vi "Set Enum String Value_csm.vi"(8 "error in (no error)":errorcluster, 9 "String Value":string, 10 "Default Enum Value":variant) -> (0 "error out":errorcluster, 2 "Enum":variant)   [LabVIEW 2017, in "Communicable State Machine.lvlib"]
doc: "Sets an enum's integer value to the position within the enum's strings matching the <B>String Value</B> input. Returns<B> Default Enum Value</B> if an error occurs."
uses:
  Communicable State Machine.lvlib
panel:
  # "[OpenG VI Tags] ***Do Not Remove***"
  # "Set Enum String Value.vi\n\nSets an enum's integer value to the position within the enum's strings matching \n\nPlease visit http://www.OpenG.org to learn about the\nOpen Source LabVIEW software movement.\n\nNOTICE -- YOU MUST LEAVE THIS NOTICE IN PLACE.  PER THE TERMS OF THE LICENSE BELOW, YOU MAY SUBLICENSE THIS SOFTWARE \nIN ANY WAY THAT DOES NOT CONFLICT WITH THIS LICENSE.\n\n### BSD License (http://www.opensource.org/licenses/bsd-license.php) Begin ###\n \nCopyright (c) 2002, Jean-Pierre Drolet <drolet_jp@hotmail.com>\nCopyright (c) 2002-2006, Jim Kring <jim@jimkring.com>\n\nAll rights reserved.\n\nRedistribution and use in source and binary forms, with or without modification, are permitted provided that the following conditions are met:\n\n    * Redistributions of source code must retain the above copyright notice, this list of conditions and the following disclaimer.\n    * Redistributions in binary form must reproduce the above copyright notice, this list of conditions and the following disclaimer in the \n       documentation and/or other materials provided with the distribution.\n    * Neither the name of SciWare, James Kring, Inc., nor the names of its contributors may be used to endorse or promote products derived \n       from this software without specific prior written permission.\n\nTHIS SOFTWARE IS PROVIDED BY THE COPYRIGHT HOLDERS AND CONTRIBUTORS \"AS IS\" AND ANY EXPRESS OR IMPLIED WARRANTIES, \nINCLUDING, BUT NOT LIMITED TO, THE IMPLIED WARRANTIES OF MERCHANTABILITY AND FITNESS FOR A PARTICULAR PURPOSE ARE \nDISCLAIMED. IN NO EVENT SHALL THE COPYRIGHT OWNER OR CONTRIBUTORS BE LIABLE FOR ANY DIRECT, INDIRECT, INCIDENTAL,\n SPECIAL, EXEMPLARY, OR CONSEQUENTIAL DAMAGES (INCLUDING, BUT NOT LIMITED TO, PROCUREMENT OF SUBSTITUTE GOODS OR \nSERVICES; LOSS OF USE, DATA, OR PROFITS; OR BUSINESS INTERRUPTION) HOWEVER CAUSED AND ON ANY THEORY OF LIABILITY, \nWHETHER IN CONTRACT, STRICT LIABILITY, OR TORT (INCLUDING NEGLIGENCE OR OTHERWISE) ARISING IN ANY WAY OUT OF THE USE \nOF THIS SOFTWARE, EVEN IF ADVISED OF THE POSSIBILITY OF SUCH DAMAGE.\n\n### BSD License End ###"
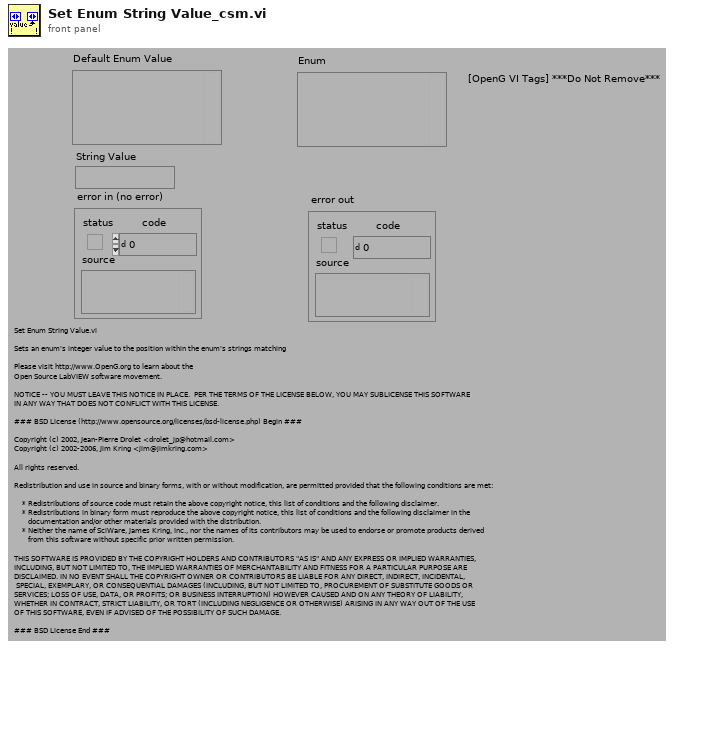
[diagram p1: front panel]
types:
  T1 = cluster{"length":u16, "private":u8, "type":enum8{"<Null>", "I8", "I16", "I32", "I64", "U8", "U16", "U32", "U64", "SGL", "DBL", "EXT", "CSG", "CDB", "CXT", "0x0F", "0x10", "0x11", "0x12", "0x13", "0x14", "Enum U8", "Enum U16", "Enum U32", "Enum U64", "SGL PQ", "DBL PQ", "EXT PQ", "CSG PQ", "CDB PQ", "CXT PQ", "0x1F", "0x20", "Boolean", "0x22", "0x23", "0x24", "0x25", "0x26", "0x27", "0x28", "0x29", "0x2A", "0x2B", "0x2C", "0x2D", "0x2E", "0x2F", "String", "0x31", "Path", "Pict", "0x34", "0x35", "0x36", "DAQ", "0x38", "0x39", "0x3A", "0x3B", "0x3C", "0x3D", "0x3E", "0x3F", "Array", "0x41", "0x42", "0x43", "0x44", "0x45", "0x46", "0x47", "0x48", "0x49", "0x4A", "0x4B", "0x4C", "0x4D", "0x4E", "0x4F", "Cluster", "0x51", "0x52", "Variant", "Waveform", "0x55", "0x56", "0x57", "0x58", "0x59", "0x5A", "0x5B", "0x5C", "0x5D", "0x5E", "Fixed Point", "0x60", "0x61", "0x62", "0x63", "0x64", "0x65", "0x66", "0x67", "0x68", "0x69", "0x6A", "0x6B", "0x6C", "0x6D", "0x6E", "0x6F", "Refnum", "0x71", "0x72", "Set Collection", "Map Collection"}, "# elements":u16}
  T2 = enum8{"<Null>", "I8", "I16", "I32", "I64", "U8", "U16", "U32", "U64", "SGL", "DBL", "EXT", "CSG", "CDB", "CXT", "0x0F", "0x10", "0x11", "0x12", "0x13", "0x14", "Enum U8", "Enum U16", "Enum U32", "Enum U64", "SGL PQ", "DBL PQ", "EXT PQ", "CSG PQ", "CDB PQ", "CXT PQ", "0x1F", "0x20", "Boolean", "0x22", "0x23", "0x24", "0x25", "0x26", "0x27", "0x28", "0x29", "0x2A", "0x2B", "0x2C", "0x2D", "0x2E", "0x2F", "String", "0x31", "Path", "Pict", "0x34", "0x35", "0x36", "DAQ", "0x38", "0x39", "0x3A", "0x3B", "0x3C", "0x3D", "0x3E", "0x3F", "Array", "0x41", "0x42", "0x43", "0x44", "0x45", "0x46", "0x47", "0x48", "0x49", "0x4A", "0x4B", "0x4C", "0x4D", "0x4E", "0x4F", "Cluster", "0x51", "0x52", "Variant", "Waveform", "0x55", "0x56", "0x57", "0x58", "0x59", "0x5A", "0x5B", "0x5C", "0x5D", "0x5E", "Fixed Point", "0x60", "0x61", "0x62", "0x63", "0x64", "0x65", "0x66", "0x67", "0x68", "0x69", "0x6A", "0x6B", "0x6C", "0x6D", "0x6E", "0x6F", "Refnum", "0x71", "0x72", "Set Collection", "Map Collection"}
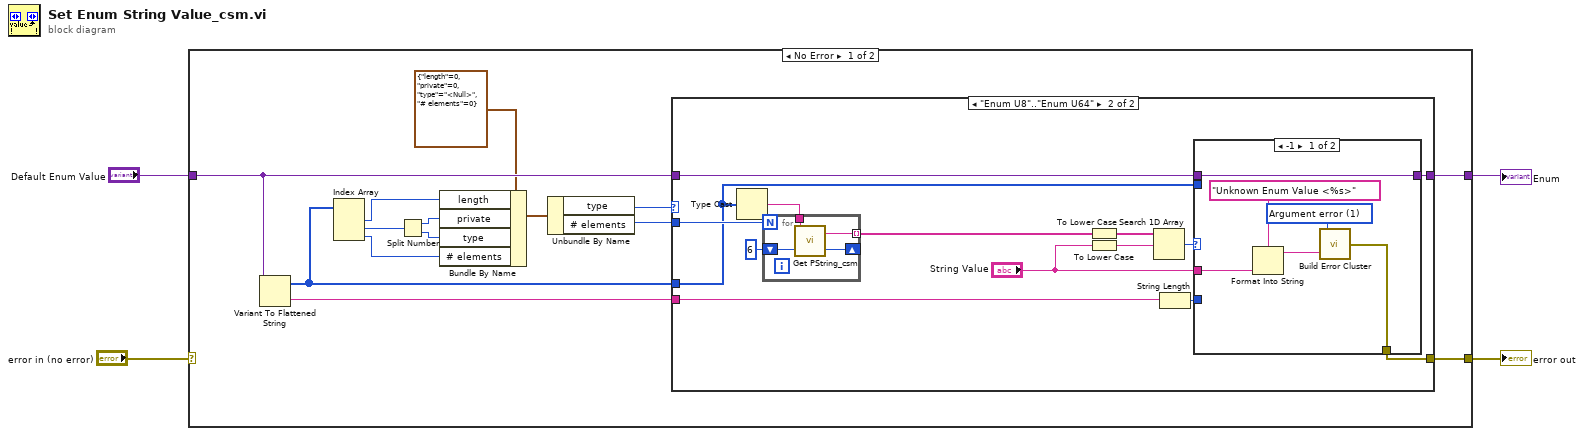
[diagram p0: block diagram]
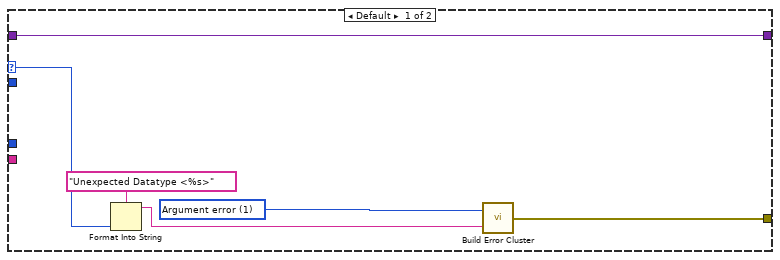
[diagram p2: hidden frame]
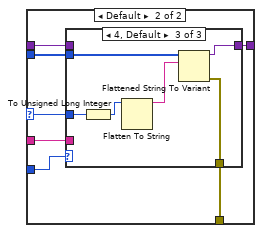
[diagram p3: hidden frame]
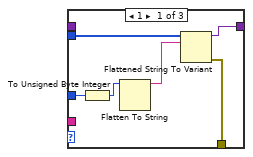
[diagram p4: hidden frame]
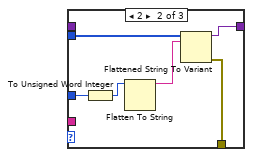
[diagram p5: hidden frame]
diagram:
  n1 = case shown="No Error" "error in (no error)" {
    selector: "error in (no error)" -> [_ w75]
    tunnel: [w18 w75] -> w4
    tunnel: [w12 w74] -> w2
    tunnel: "Default Enum Value" -> [w11 w74]
    frame No Error {
      n2 = Variant To Flattened String(Variant=w11) -> (data string=w14:string, 1:w15:i16[])
      n3 = Index Array(array=w15) -> (element #1=w6:i16, element #2=w9:i16, element #3=w10:i16)  [unwired: 3 in]
      n4 = Split Number(x=w9) -> (hi(x)=w7:u8, lo(x)=w8:u8)
      n5 = Bundle By Name(cluster=T1 {"length"=0, "private"=0, "type"=enum."<Null>", "# elements"=0} ("Type Descriptor Header"), "length"=w6, "private"=w7, "type"=w8, "# elements"=w10) -> (w17:T1)
      n6 = Unbundle By Name(w17) -> ("type"=w16:T2, "# elements"=w13:u16)
      n7 = case shown="\"Enum U8\"..\"Enum U64\"" w16 {
        selector: w16 -> [w21 _]
        tunnel: [w24 w29] -> w18
        tunnel: w15 -> [_ w30]
        tunnel: w14 -> [_ w33]
        tunnel: w13 -> [_ w36]
        tunnel: [w22 w31] -> w12
        tunnel: w11 -> [w22 w32]
        frame Default {
          w23 = 1 items=["No error", "Argument error", "Memory is full", "Out of zone", "End of file", "File already open", "Generic file I/O error", "File not found", "File permission error", "Disk is full", "Duplicate path", "Too many files open", "System feature not enabled", "Resource file not found", "Cannot add resource", "Resource not found", "Image not found", "Image memory error", "Pen does not exist", "Config type invalid", "Config token not found", "Config parse error", "Config memory error", "Bad external code format", "Bad external code offset", "External code not present", "Null window", "Destroy window error", "Null menu", "Print aborted", "Bad print record", "Print driver error", "Windows error during printing", "Memory error during printing", "Print dialog error", "Generic print error", "Invalid device refnum", "Device not found", "Device parameter error", "Device unit error", "Cannot open device", "Device call aborted", "Generic error", "Cancelled by user", "Object ID too low", "Object ID too high", "Object not in heap", "Unknown heap", "Unknown object (invalid DefProc)", "Unknown object (DefProc not in table)", "Message out of range", "Invalid (null) method", "Unknown message", "Manager call not supported", "Bad address", "Network operation in progress", "Network operation timed out", "Connection is busy", "Network attribute not supported", "Network error", "Address in use", "System out of memory", "Connection aborted", "Connection refused", "Not connected", "Already connected", "Connection closed", "Initialization error (interapplication manager)", "Bad occurrence", "Wait on unbound occurrence handler", "Occurrence queue overflow", "Datalog type conflict", "Unused", "Unrecognized type (interapplication manager)", "Memory corrupt", "Failed to make temporary DLL", "Old CIN version", "Drag socket not found", "Failed to load drop-object", "Failed to register OLE object", "Failed to release OLE object", "Format specifier type mismatch", "Unknown format specifier", "Too few format specifiers", "Too many format specifiers", "Scan failed", "Newer CIN version", "Error converting to variant", "Runtime menu error", "Password tampered", "Variant attribute not found", "Incompatible variant data type", "Event data is not available", "Event Store is not present", "Occurrence is not found", "Event Queue is not created", "Event info is not available", "Refnum passed is NULL", "Error retrieving Class GUID", "Error retrieving CoClass GUID", "Error retrieving TypeLib GUID.", "Bad built application magic bytes.", "Specific driver is different from the specific driver associated with the Logical Name.", "There is no session opened to the class driver.", "Max Error", "MAX - Error with config objects", "MAX - Error loading configuration", "MAX - Group not supported"]
          n8 = Format Into String(format string="Unexpected Datatype <%s>" ("Format String"), w21) -> (resulting string=w19:string)  [unwired: 2 in, 1 out]
          n9 = call "Build Error Cluster.vi"("String to Prepend to Source (\"\")"=w19, "Code"=w23) -> ("error out"=w24:errorcluster)
        }
        frame "Enum U8".."Enum U64" {
          n10 = Type Cast(x=w30) -> (*(type *) &x=w35:string)  [unwired: 1 in]
          n11 = for {
            N: w36 -> [_]
            tunnel: w35 -> [w71]
            shift-right: [w72] -> _
            shift-left: 6 -> [w73]
            tunnel: [w70] -> w34 mode=indexing
            n12 = call "Get PString_csm.vi"("Offset (0)"=w73, "String"=w71) -> ("Offset Past PString"=w72:i32, "PString"=w70:string)
          }
          n13 = To Lower Case(string=w34) -> (all lower case string=w25:string[])
          n14 = To Lower Case(string="String Value") -> (all lower case string=w26:string)
          n15 = Search 1D Array(1D array=w25, element=w26) -> (index of element=w27:i32)  [unwired: 1 in]
          n16 = String Length(string=w33) -> (length=w37:i32)
          n17 = case shown="-1" w27 {
            selector: w27 -> [_ w45]
            tunnel: w37 -> [_ w51]
            tunnel: w32 -> [w44 w50]
            tunnel: [w44 w49] -> w31
            tunnel: w30 -> [_ w48]
            tunnel: [w39 w47] -> w29
            tunnel: "String Value" -> [w40 w46]
            frame -1 {
              w43 = 1 items=["No error", "Argument error", "Memory is full", "Out of zone", "End of file", "File already open", "Generic file I/O error", "File not found", "File permission error", "Disk is full", "Duplicate path", "Too many files open", "System feature not enabled", "Resource file not found", "Cannot add resource", "Resource not found", "Image not found", "Image memory error", "Pen does not exist", "Config type invalid", "Config token not found", "Config parse error", "Config memory error", "Bad external code format", "Bad external code offset", "External code not present", "Null window", "Destroy window error", "Null menu", "Print aborted", "Bad print record", "Print driver error", "Windows error during printing", "Memory error during printing", "Print dialog error", "Generic print error", "Invalid device refnum", "Device not found", "Device parameter error", "Device unit error", "Cannot open device", "Device call aborted", "Generic error", "Cancelled by user", "Object ID too low", "Object ID too high", "Object not in heap", "Unknown heap", "Unknown object (invalid DefProc)", "Unknown object (DefProc not in table)", "Message out of range", "Invalid (null) method", "Unknown message", "Manager call not supported", "Bad address", "Network operation in progress", "Network operation timed out", "Connection is busy", "Network attribute not supported", "Network error", "Address in use", "System out of memory", "Connection aborted", "Connection refused", "Not connected", "Already connected", "Connection closed", "Initialization error (interapplication manager)", "Bad occurrence", "Wait on unbound occurrence handler", "Occurrence queue overflow", "Datalog type conflict", "Unused", "Unrecognized type (interapplication manager)", "Memory corrupt", "Failed to make temporary DLL", "Old CIN version", "Drag socket not found", "Failed to load drop-object", "Failed to register OLE object", "Failed to release OLE object", "Format specifier type mismatch", "Unknown format specifier", "Too few format specifiers", "Too many format specifiers", "Scan failed", "Newer CIN version", "Error converting to variant", "Runtime menu error", "Password tampered", "Variant attribute not found", "Incompatible variant data type", "Event data is not available", "Event Store is not present", "Occurrence is not found", "Event Queue is not created", "Event info is not available", "Refnum passed is NULL", "Error retrieving Class GUID", "Error retrieving CoClass GUID", "Error retrieving TypeLib GUID.", "Bad built application magic bytes.", "Specific driver is different from the specific driver associated with the Logical Name.", "There is no session opened to the class driver.", "Max Error", "MAX - Error with config objects", "MAX - Error loading configuration", "MAX - Group not supported"]
              n18 = Format Into String(format string="Unknown Enum Value <%s>" ("Format String"), w40) -> (resulting string=w42:string)  [unwired: 2 in, 1 out]
              n19 = call "Build Error Cluster.vi"("String to Prepend to Source (\"\")"=w42, "Code"=w43) -> ("error out"=w39:errorcluster)
            }
            frame Default {
              n20 = case shown="4, Default" w51 {
                tunnel: w45 -> [w57 w63 w69]
                tunnel: w50 -> [_ _ _]
                tunnel: [w53 w59 w65] -> w49
                tunnel: w48 -> [w55 w61 w67]
                tunnel: [w52 w58 w64] -> w47
                tunnel: w46 -> [_ _ _]
                frame 1 {
                  n21 = To Unsigned Byte Integer(number=w57) -> (unsigned 8bit integer=w56:u8)
                  n22 = Flatten To String(anything=w56) -> (data string=w54:string)  [unwired: 3 in, 2 out]
                  n23 = Flattened String To Variant(6:w54, 7:w55) -> (0:w52:errorcluster, 3:w53:variant)  [unwired: 1 in]
                }
                frame 2 {
                  n24 = To Unsigned Word Integer(number=w63) -> (unsigned 16bit integer=w62:u16)
                  n25 = Flatten To String(anything=w62) -> (data string=w60:string)  [unwired: 3 in, 2 out]
                  n26 = Flattened String To Variant(6:w60, 7:w61) -> (0:w58:errorcluster, 3:w59:variant)  [unwired: 1 in]
                }
                frame 4, Default {
                  n27 = To Unsigned Long Integer(number=w69) -> (unsigned 32bit integer=w68:u32)
                  n28 = Flatten To String(anything=w68) -> (data string=w66:string)  [unwired: 3 in, 2 out]
                  n29 = Flattened String To Variant(6:w66, 7:w67) -> (0:w64:errorcluster, 3:w65:variant)  [unwired: 1 in]
                }
              }
            }
          }
        }
      }
    }
    frame Error {
    }
  }
  "error out" <- w4
  "Enum" <- w2
